vi "Station Reset.vi"(8 "error in (no error)":errorcluster, 11 "Station in":refnum<class "Station.lvclass">) -> (0 "error out":errorcluster, 3 "Station out":refnum<class "Station.lvclass">)   [LabVIEW 2018, in "Station.lvclass"]
uses:
  Station.lvclass
  Station Support/Controls/Server Control.ctl
  Station.lvclass/Station.ctl
panel:
  out "Currently Resetting Instrument:":string
  # "Model Number:\nInstrument Number:\nRack ID:\nInst Mnemonic:\nComp Mnemonic:\nSubsys Mnemonic:\nIP Address:\nSub Address:\nFirmware Rev:\nExpected Options:\nRequired Options: \nExcluded Options:"
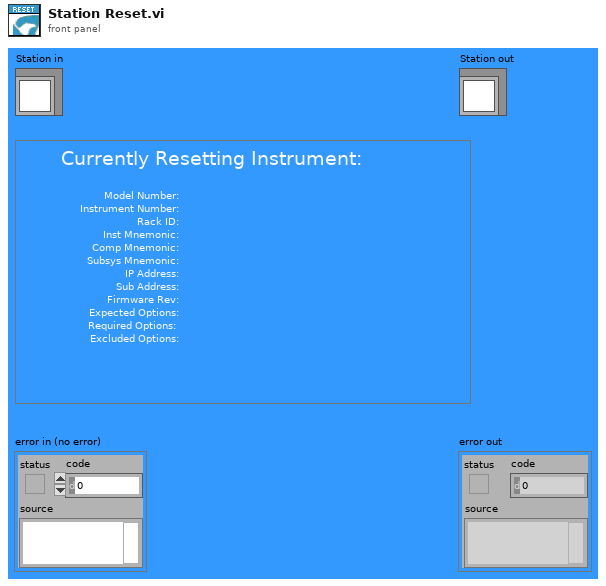
[diagram p1: front panel]
types:
  T1 = typedef "Server Control.ctl" = enum16{"Open New Reference", "Remove Reference", "Kill Server", "Set Station Ref", "Get Station Ref"}
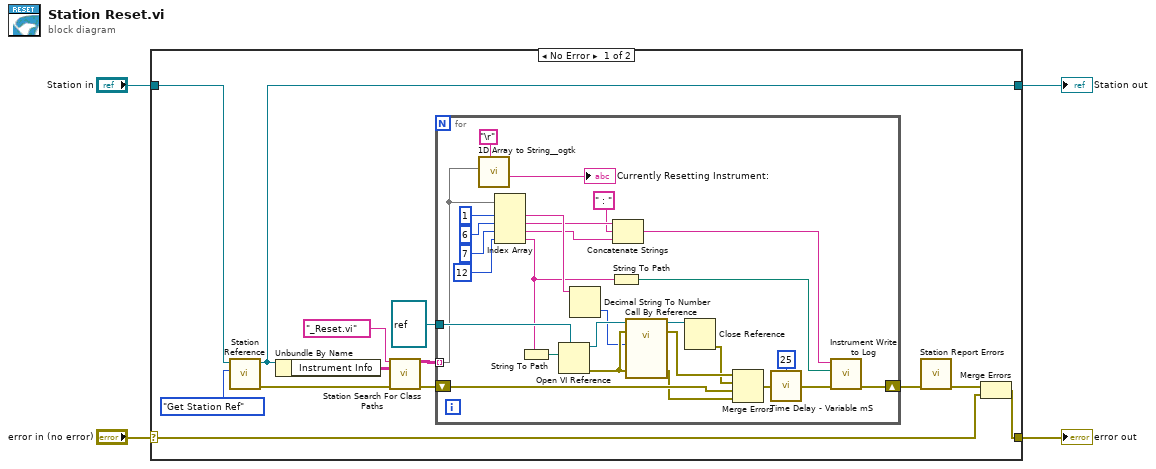
[diagram p0: block diagram]
diagram:
  n1 = case shown="No Error" "error in (no error)" {
    selector: "error in (no error)" -> [w9 w47]
    tunnel: [w11 w47] -> w4
    tunnel: "Station in" -> [w7 w46]
    tunnel: [w6 w46] -> w1
    frame No Error {
      n2 = call "Station Reference.vi"("Action (0: Create)"=Server_Control."Get Station Ref", "Station in"=w7) -> ("error out"=w8:errorcluster, "Station out"=w6:refnum<class "Station.lvclass">)  [unwired: 8 in]
      n3 = Unbundle By Name(w6) -> ("Instrument Info"=w10:string[][])
      n4 = call "Station Search For Class Paths.vi"("VI select"="_Reset.vi", "Instrument Info"=w10, "error in (no error)"=w8) -> ("Updated Inst Info"=w14:string[][], "error out"=w15:errorcluster)  [unwired: 11 in]
      n5 = for {
        tunnel: w14 -> [w34] mode=indexing
        tunnel: refnum<vi> refnum ("VI Refnum") -> [w45]
        shift-right: [w19] -> w13
        shift-left: w15 -> [w38]
        n6 = call <userlib>:"1D Array to String__ogtk.vi"("delimiter (Tab)"="\r", "Array of Strings"=w34) -> ("delimited string"=→"Currently Resetting Instrument:":string)  [unwired: 9 in]
        n7 = Index Array(array=w34, index #1=1 ("index"), index #2=6 ("index"), index #3=7 ("index"), index #4=12 ("index")) -> (element #1=w32:string, element #2=w26:string, element #3=w24:string, element #4=w27:string)
        n8 = String To Path(string=w27) -> (path=w42:path)
        n9 = Open VI Reference(type specifier VI Refnum (for type only)=w45, vi path=w42) -> (vi reference=w43:refnum<vi>, error out=w44:errorcluster)  [unwired: 4 in]
        n10 = Decimal String To Number(string=w32) -> (number=w37:i32)  [unwired: 2 in, 1 out]
        n11 = String To Path(string=w27) -> (path=w31:path)
        n12 = Concatenate Strings(w26, " : " ("string"), w24) -> (w23:string)
        n13 = call-by-ref "?"(reference=w43, error in=w44, "User Reference"=w37, "error in (no error)"=w44) -> (reference out=w40:refnum<vi>, error out=w41:errorcluster, 19:"error out"=w36:errorcluster)  [unwired: 17 in]
        n14 = Close Reference(reference=w40) -> (error out=w39:errorcluster)  [unwired: 1 in]
        n15 = Merge Errors(w41, w39, w38, w36) -> (w20:errorcluster)
        n16 = call "Time Delay - Variable mS.vi"("milliseconds to wait"=u32 25, "error in (no error)"=w20) -> ("error out"=w21:errorcluster)  [unwired: 2 in]
        n17 = call "Instrument Write to Log.vi"("error in (no error)"=w21, "Current VI's Path"=w31, "Insstrument Address"=w23) -> ("error out"=w19:errorcluster)  [unwired: 8 in]
      }
      n18 = call "Station Report Errors.vi"("error in (no error)"=w13) -> ("error out"=w12:errorcluster)  [unwired: 10 in]
      n19 = Merge Errors(w12, w9) -> (w11:errorcluster)
    }
    frame Error {
    }
  }
  "error out" <- w4
  "Station out" <- w1
